vi "FGVLateralFilter.vi"(5 "Enum":T1, 6 "error in":errorcluster, 8 "ZPK input cluster":cluster{dbl, cdb[][], cdb[][], dbl}, 9 "Filter valid input":bool) -> (0 "error out":errorcluster, 2 "ZPK input cluster 2":cluster{dbl, cdb[][], cdb[][], dbl}, 3 "Filter valid output":bool)   [LabVIEW 2016]
uses:
  controls/Enum.ctl
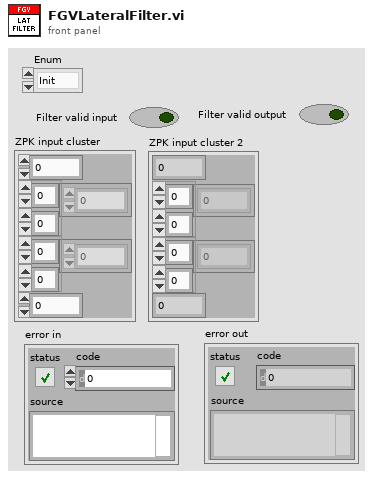
[diagram p1: front panel]
types:
  T1 = typedef "Enum.ctl" = enum16{"Init", "Read", "Write"}
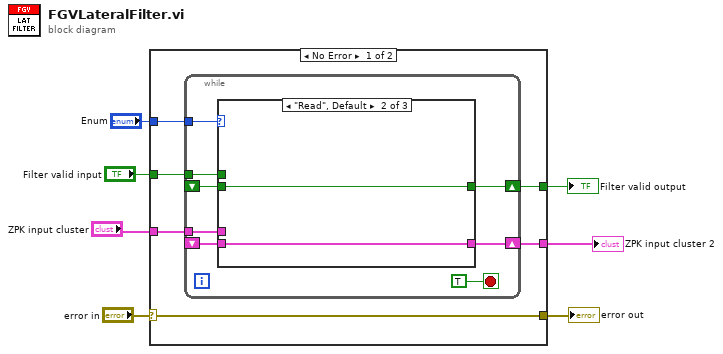
[diagram p0: block diagram]
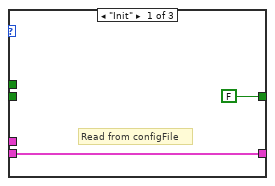
[diagram p2: hidden frame]
diagram:
  n1 = case shown="No Error" "error in" {
    selector: "error in" -> [w12 w30]
    tunnel: "Enum" -> [w13 _]
    tunnel: [w12 w30] -> w6
    tunnel: "ZPK input cluster" -> [w11 w29]
    tunnel: [w10 w29] -> w1
    tunnel: [w9 w28] -> w4
    tunnel: "Filter valid input" -> [w8 w28]
    frame No Error {
      n2 = while {
        tunnel: w13 -> [w20]
        tunnel: w11 -> [w19]
        shift-right: [w18] -> w10
        shift-left: _ -> [w17]
        shift-right: [w16] -> w9
        shift-left: _ -> [w15]
        tunnel: w8 -> [w14]
        stop <- TRUE stop-if-true
        n3 = case shown="\"Read\", Default" w20 {
          tunnel: w19 -> [_ _ w27]
          tunnel: [w23 w25 w27] -> w18
          tunnel: w17 -> [w23 w25 _]
          tunnel: [FALSE w24 w26] -> w16
          tunnel: w15 -> [_ w24 _]
          tunnel: w14 -> [_ _ w26]
          frame "Init" {
            # "Read from configFile"
          }
          frame "Read", Default {
          }
          frame "Write" {
          }
        }
      }
    }
    frame Error {
    }
  }
  "error out" <- w6
  "Filter valid output" <- w4
  "ZPK input cluster 2" <- w1
